vi "Matrix_Pow.vi"(10 "Exponent":dbl, 11 "input matrix":T1) -> (0 "Error":bool, 3 "output matrix":T1, 4 "ExponentNotRational":bool)   [LabVIEW 2019, in "Trajectory_Library.lvlib"]
doc: "Creates a new LINEAR SYSTEM data cluster with the specified values. \n\n\nInputs: \n - XXX -- XXX.\n\nOutputs:\n - XXX -- XXX."
uses:
  Trajectory_Library.lvlib
  <vilib>/Analysis/Matrix/Datatypes/RealMatrix.ctl
  <vilib>/Analysis/7linalg.llb/Real Matrix Power.vi
  <vilib>/Analysis/NI_AALBase.lvlib
  <vilib>/Analysis/Matrix/NI_Matrix.lvlib
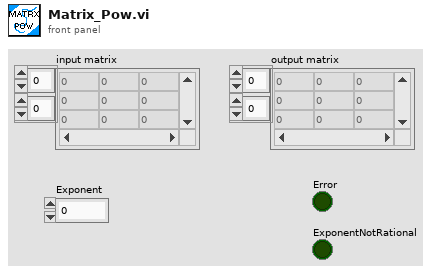
[diagram p1: front panel]
types:
  T1 = typedef "NI_Matrix.lvlib/RealMatrix.ctl" = dbl[][]
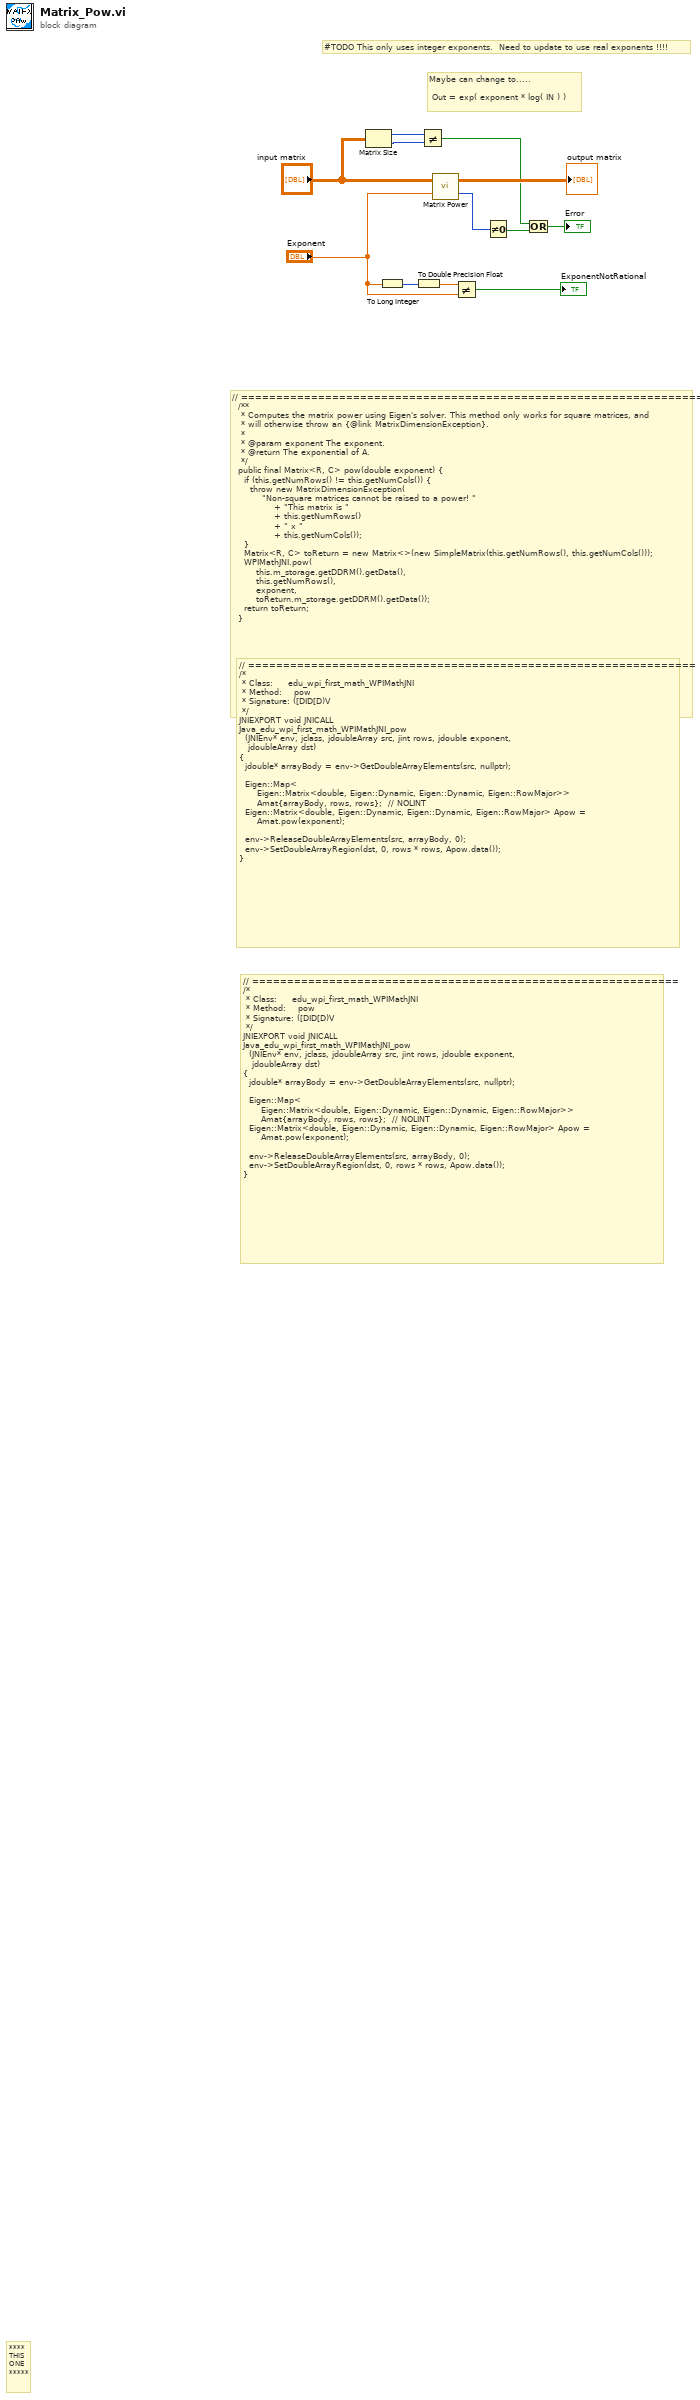
[diagram p0: block diagram]
diagram:
  # "// =============================================================\n/*\n * Class:     edu_wpi_first_math_WPIMathJNI\n * Method:    pow\n * Signature: ([DID[D)V\n */\nJNIEXPORT void JNICALL\nJava_edu_wpi_first_math_WPIMathJNI_pow\n  (JNIEnv* env, jclass, jdoubleArray src, jint rows, jdouble exponent,\n   jdoubleArray dst)\n{\n  jdouble* arrayBody = env->GetDoubleArrayElements(src, nullptr);\n\n  Eigen::Map<\n      Eigen::Matrix<double, Eigen::Dynamic, Eigen::Dynamic, Eigen::RowMajor>>\n      Amat{arrayBody, rows, rows};  // NOLINT\n  Eigen::Matrix<double, Eigen::Dynamic, Eigen::Dynamic, Eigen::RowMajor> Apow =\n      Amat.pow(exponent);\n\n  env->ReleaseDoubleArrayElements(src, arrayBody, 0);\n  env->SetDoubleArrayRegion(dst, 0, rows * rows, Apow.data());\n}"
  # "// ================================================================\n/*\n * Class:     edu_wpi_first_math_WPIMathJNI\n * Method:    pow\n * Signature: ([DID[D)V\n */\nJNIEXPORT void JNICALL\nJava_edu_wpi_first_math_WPIMathJNI_pow\n  (JNIEnv* env, jclass, jdoubleArray src, jint rows, jdouble exponent,\n   jdoubleArray dst)\n{\n  jdouble* arrayBody = env->GetDoubleArrayElements(src, nullptr);\n\n  Eigen::Map<\n      Eigen::Matrix<double, Eigen::Dynamic, Eigen::Dynamic, Eigen::RowMajor>>\n      Amat{arrayBody, rows, rows};  // NOLINT\n  Eigen::Matrix<double, Eigen::Dynamic, Eigen::Dynamic, Eigen::RowMajor> Apow =\n      Amat.pow(exponent);\n\n  env->ReleaseDoubleArrayElements(src, arrayBody, 0);\n  env->SetDoubleArrayRegion(dst, 0, rows * rows, Apow.data());\n}"
  # "Maybe can change to.....\n\n Out = exp( exponent * log( IN ) )"
  # "#TODO This only uses integer exponents.  Need to update to use real exponents !!!!"
  # "// ===================================================================\n  /**\n   * Computes the matrix power using Eigen's solver. This method only works for square matrices, and\n   * will otherwise throw an {@link MatrixDimensionException}.\n   *\n   * @param exponent The exponent.\n   * @return The exponential of A.\n   */\n  public final Matrix<R, C> pow(double exponent) {\n    if (this.getNumRows() != this.getNumCols()) {\n      throw new MatrixDimensionException(\n          \"Non-square matrices cannot be raised to a power! \"\n              + \"This matrix is \"\n              + this.getNumRows()\n              + \" x \"\n              + this.getNumCols());\n    }\n    Matrix<R, C> toReturn = new Matrix<>(new SimpleMatrix(this.getNumRows(), this.getNumCols()));\n    WPIMathJNI.pow(\n        this.m_storage.getDDRM().getData(),\n        this.getNumRows(),\n        exponent,\n        toReturn.m_storage.getDDRM().getData());\n    return toReturn;\n  }"
  # "****\nTHIS\nONE\n*****"
  n1 = Matrix Size(0:"input matrix") -> (1:w9:i32, 2:w8:i32)
  n2 = To Long Integer(number="Exponent") -> (32bit integer=w4:i32)
  n3 = To Double Precision Float(number=w4) -> (double precision float=w3:dbl)
  n4 = Not Equal?(x=w9, y=w8) -> (x != y?=w5:bool)
  n5 = call-poly <vilib>:"Matrix Power.vi"("n"="Exponent", "Input Matrix"="input matrix") -> ("error"=w11:i32, "Matrix Power"=→"output matrix":T1)
  n6 = Not Equal?(x=w3, y="Exponent") -> (x != y?=→"ExponentNotRational":bool)
  n7 = Not Equal To 0?(x=w11) -> (x != 0?=w6:bool)
  n8 = Or(x=w5, y=w6) -> (x .or. y?=→"Error":bool)
